vi "SetCurrentScreen.vi"(8 "error in (no error)":errorcluster, 11 "SnakeGame in":refnum<class "SnakeGame.lvclass">) -> (0 "error out":errorcluster, 3 "SnakeGame out":refnum<class "SnakeGame.lvclass">)   [LabVIEW 2019, in "RT_Game.lvlib" / "SnakeGame.lvclass"]
uses:
  SnakeGame.lvclass
  SnakeGame.lvclass/SnakeGame.ctl
  Game/Game.lvclass
  Engine/Engine.lvclass
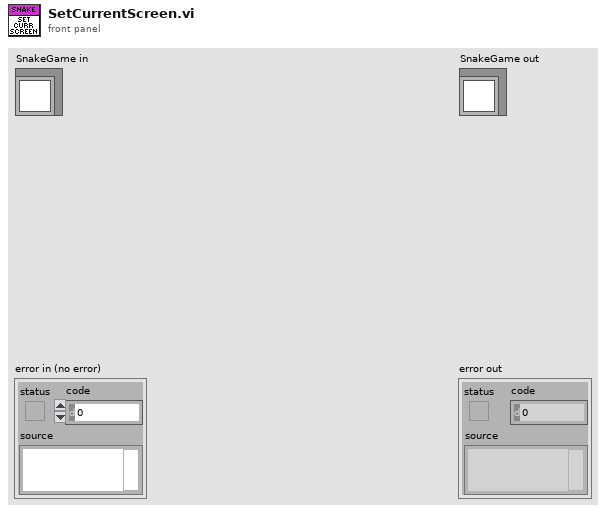
[diagram p1: front panel]
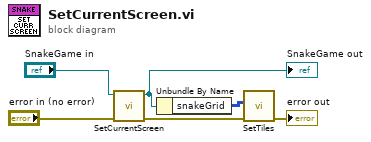
[diagram p0: block diagram]
diagram:
  n1 = call-parent "SetCurrentScreen.vi"("error in (no error)"="error in (no error)", "Game in"="SnakeGame in") -> ("error out"=w4:errorcluster, "Game out"=w1:refnum<class "SnakeGame.lvclass">)  [unwired: 8 in]
  "SnakeGame out" <- w1
  n2 = Unbundle By Name(w1) -> ("snakeGrid"=w2:u32[][])
  n3 = call "SetTiles.vi"("error in (no error)"=w4, "TileCodes"=w2) -> ("error out"=→"error out":errorcluster)  [unwired: 9 in]
